vi "GetElements.vi"(8 "error in (no error)":errorcluster, 11 "Collection in":refnum<class "Collection.lvclass">) -> (0 "error out":errorcluster, 2 "Elements":refnum<class "IRenderable.lvclass">[](array[class]), 3 "Collection out":refnum<class "Collection.lvclass">)   [LabVIEW 2021, in "LvMarkdown.lvlib" / "Collection.lvclass"]
uses:
  Collection.lvclass
  Collection.lvclass/Collection.ctl
  IRenderable/IRenderable.lvclass
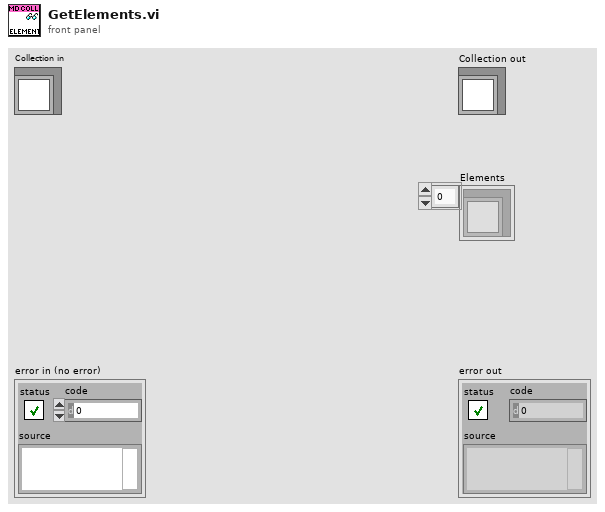
[diagram p1: front panel]
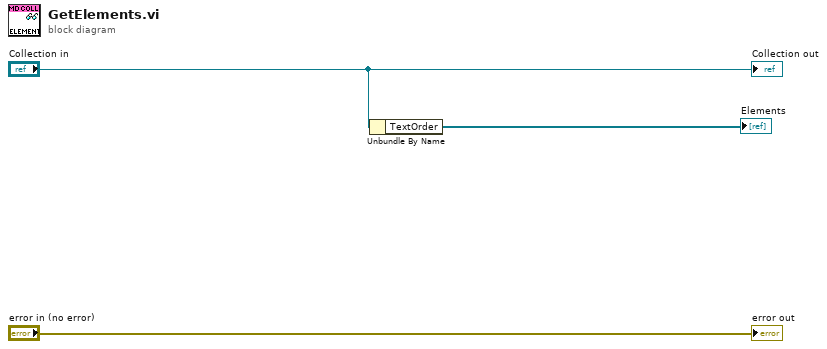
[diagram p0: block diagram]
diagram:
  n1 = Unbundle By Name("Collection in") -> ("TextOrder"=→"Elements":refnum<class "IRenderable.lvclass">[])
  "error out" <- "error in (no error)"
  "Collection out" <- "Collection in"
